vi "Split Timestamp and Log.vi"(8 "error in (no error)":errorcluster, 11 "Array":string[](array[string])) -> (0 "error out":errorcluster, 3 "Split String":string[][](array[string]))   [LabVIEW 2019]
doc: "Given a 1D array of the format \"TIMESTAMP LOG\", return a 2D array where each 1D array is in the format TIMESTAMP, LOG."
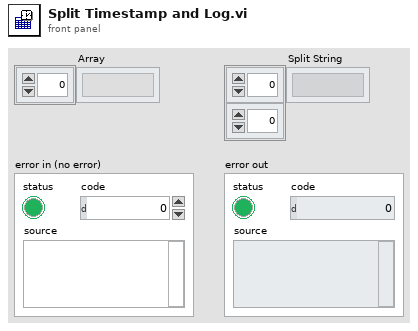
[diagram p1: front panel]
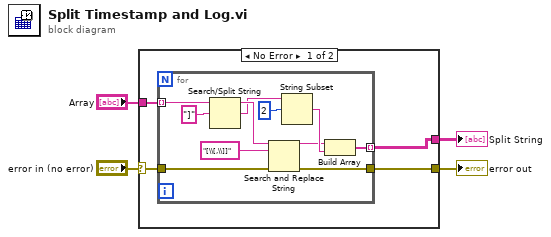
[diagram p0: block diagram]
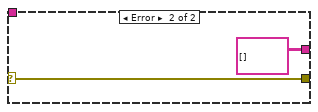
[diagram p2: hidden frame]
diagram:
  n1 = case shown="No Error" "error in (no error)" {
    selector: "error in (no error)" -> [w7 w21]
    tunnel: [w8 string[][] [] ("Split String")] -> w2
    tunnel: [w6 w21] -> w3
    tunnel: "Array" -> [w5 _]
    frame No Error {
      n2 = for {
        tunnel: w7 -> [w14]
        tunnel: [w13] -> w8 mode=indexing
        tunnel: [w18] -> w6
        tunnel: w5 -> [w16] mode=indexing
        n3 = Search/Split String(string=w16, search string/char (-)="]") -> (substring before match=w15:string, match + rest of string=w12:string)  [unwired: 1 in, 1 out]
        n4 = Search and Replace String(input string=w15, search string="[\\[,\\]]", error in=w14) -> (result string=w9:string, error out=w18:errorcluster)  [unwired: 5 in, 2 out]
        n5 = String Subset(string=w12, offset (0)=2) -> (substring=w10:string)  [unwired: 1 in]
        n6 = Build Array(w9, w10) -> (w13:string[])
      }
    }
    frame Error {
    }
  }
  "error out" <- w3
  "Split String" <- w2
